vi "AssembleBLMultiplotScript-Spectra.vi"(0 "gnuplotIn":string, 5 "SpectrumFilename":string="spec.dat", 9 "f.E(f) Bounds":T1={"Min"={"Auto"=FALSE, "Value"=5.0}, "Max"={"Auto"=FALSE, "Value"=2000.0}}, 12 "f Bounds":T1={"Min"={"Auto"=FALSE, "Value"=0.0}, "Max"={"Auto"=FALSE, "Value"=1.2}}) -> (4 "gnuplotOut":string)   [LabVIEW 2013]
uses:
  minAndMax.ctl
  AutoManualNumber.ctl
  axisName.ctl
  ticsAndGrids.ctl
  tics.ctl
  grids.ctl
  legendProperties.ctl
  legendAppearance.ctl
  alignment.ctl
  at.ctl
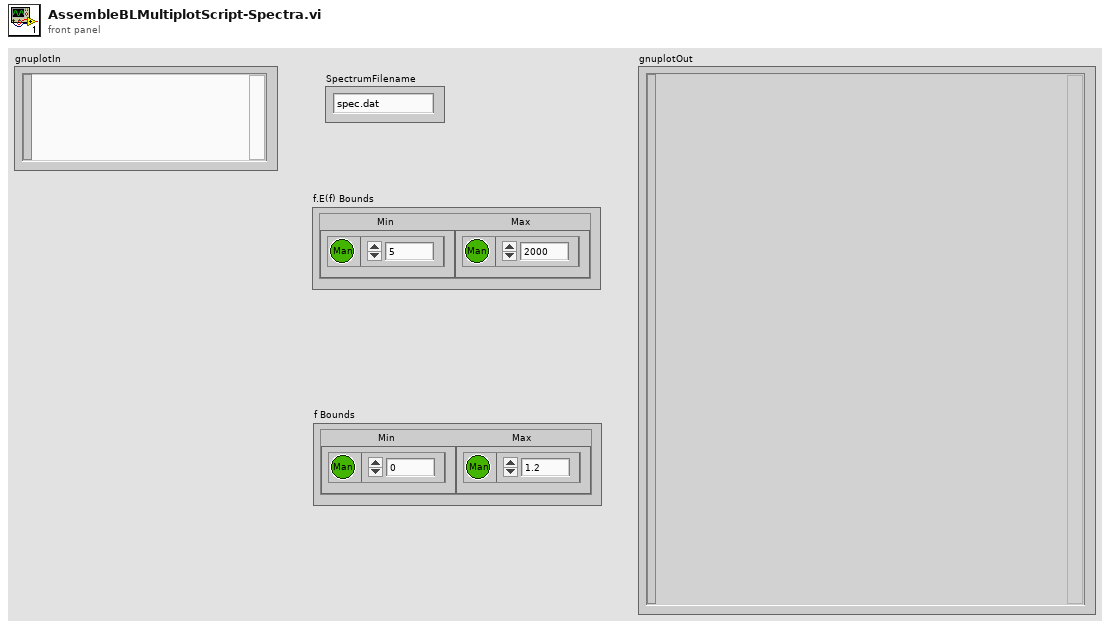
[diagram p1: front panel]
types:
  T1 = typedef "minAndMax.ctl" = cluster{"Min":T2, "Max":T2}
  T2 = typedef "AutoManualNumber.ctl" = cluster{"Auto":bool, "Value":dbl}
  T3 = typedef "legendProperties.ctl" = cluster{"Appearance":T4, "Alignment":T5, "Location":string, "\"At\" location":T6}
  T4 = typedef "legendAppearance.ctl" = cluster{"layout":string, "text-sample order":string, "key order":string, "surroundingBox":string}
  T5 = typedef "alignment.ctl" = cluster{"Horizontal":string, "Vertical":string}
  T6 = typedef "at.ctl" = cluster{"XcoordSys":string, "YcoordSys":string, "Xvalue":dbl, "Yvalue":dbl}
  T7 = typedef "ticsAndGrids.ctl" = cluster{"tics":T8, "Grids":T9, "Mapping":enum8{"Lin", "Log"}}
  T8 = typedef "tics.ctl" = cluster{"ticMin":dbl, "ticStep":dbl, "ticMax":dbl, "minorDivsPerMajor":i32, "ticSpacing":enum16{"Auto Tics", "Fixed spacing", "Fixed Minimum and Spacing", "Start, Spacing and Maximum", "Approx n Tics (rounded)"}, "ticPosition":enum16{"Inside, no mirror", "Inside, mirrored", "Outside, no mirror", "Outside, mirrored", "Invisible"}}
  T9 = typedef "grids.ctl" = cluster{"Gridlines":enum16{"No grids", "Major grid", "Minor grid", "Major and Minor"}, "Zeroaxis":enum16{"No zero axis", "Show zero axis"}}
  T10 = typedef "axisName.ctl" = string
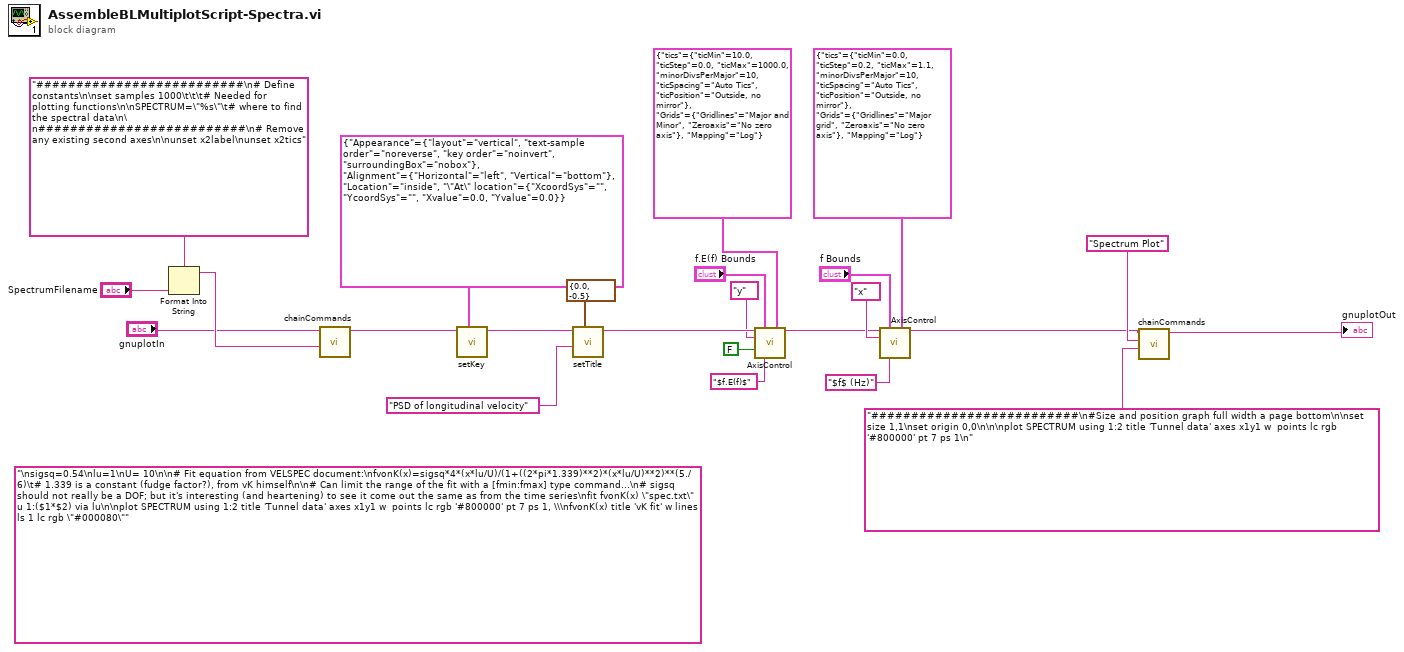
[diagram p0: block diagram]
diagram:
  (unwired) "\nsigsq=0.54\nlu=1\nU= 10\n\n# Fit equation from VELSPEC document:\nfvonK(x)=sigsq*4*(x*lu/U)/(1+((2*pi*1.339)**2)*(x*lu/U)**2)**(5./6)\t# 1.339 is a constant (fudge factor?), from vK himself\n\n# Can limit the range of the fit with a [fmin:fmax] type command...\n# sigsq should not really be a DOF; but it's interesting (and heartening) to see it come out the same as from the time series\nfit fvonK(x) \"spec.txt\" u 1:($1*$2) via lu\n\nplot SPECTRUM using 1:2 title 'Tunnel data' axes x1y1 w  points lc rgb '#800000' pt 7 ps 1, \\\nfvonK(x) title 'vK fit' w lines ls 1 lc rgb \"#000080\""
  n1 = Format Into String(format string="##########################\n# Define constants\n\nset samples 1000\t\t\t# Needed for plotting functions\n\nSPECTRUM=\"%s\"\t# where to find the spectral data\n\n##########################\n# Remove any existing second axes\n\nunset x2label\nunset x2tics" ("Command"), "SpectrumFilename") -> (resulting string=w13:string)  [unwired: 2 in, 1 out]
  n2 = call "chainCommands.vi"("Command"=w13, "StringIn"="gnuplotIn") -> ("StringOut"=w11:string)  [unwired: 9 in]
  n3 = call "setKey.vi"("LegendProperties"=T3 {"Appearance"={"layout"="vertical", "text-sample order"="noreverse", "key order"="noinvert", "surroundingBox"="nobox"}, "Alignment"={"Horizontal"="left", "Vertical"="bottom"}, "Location"="inside", "\"At\" location"={"XcoordSys"="", "YcoordSys"="", "Xvalue"=0.0, "Yvalue"=0.0}}, "String in"=w11) -> ("String out"=w24:string)  [unwired: 8 in, 1 out]
  n4 = call "setTitle.vi"("Offset"=cluster{"horizontal":dbl, "vertical":dbl} {"horizontal"=0.0, "vertical"=-0.5}, "Title"="PSD of longitudinal velocity", "String in"=w24) -> ("String out"=w23:string)  [unwired: 7 in, 1 out]
  n5 = call "AxisControl.vi"("String in"=w23, "AxisBounds"="f.E(f) Bounds", "ticsAndGrids"=T7 {"tics"={"ticMin"=10.0, "ticStep"=0.0, "ticMax"=1000.0, "minorDivsPerMajor"=10, "ticSpacing"=enum."Auto Tics", "ticPosition"=enum."Outside, no mirror"}, "Grids"={"Gridlines"=enum."Major and Minor", "Zeroaxis"=enum."No zero axis"}, "Mapping"=enum."Log"}, "Axis"=T10 "y", "ShowNumbers?"=FALSE, "Axis Label"="$f.E(f)$") -> ("String out"=w18:string)  [unwired: 8 in, 1 out]
  n6 = call "AxisControl.vi"("String in"=w18, "AxisBounds"="f Bounds", "ticsAndGrids"=T7 {"tics"={"ticMin"=0.0, "ticStep"=0.2, "ticMax"=1.1, "minorDivsPerMajor"=10, "ticSpacing"=enum."Auto Tics", "ticPosition"=enum."Outside, no mirror"}, "Grids"={"Gridlines"=enum."Major grid", "Zeroaxis"=enum."No zero axis"}, "Mapping"=enum."Log"}, "Axis"=T10 "x", "Axis Label"="$f$ (Hz)") -> ("String out"=w3:string)  [unwired: 9 in, 1 out]
  n7 = call "chainCommands.vi"("Command"="##########################\n#Size and position graph full width a page bottom\n\nset size 1,1\nset origin 0,0\n\n\nplot SPECTRUM using 1:2 title 'Tunnel data' axes x1y1 w  points lc rgb '#800000' pt 7 ps 1\n", "Comments"="Spectrum Plot", "StringIn"=w3) -> ("StringOut"=→"gnuplotOut":string)  [unwired: 8 in]
